vi "Loop_SM.vi"() -> ()   [LabVIEW 2017, in "Claw.lvlib"]
uses:
  Claw.lvlib
  TypeDef/CLUSTER_Two Motor Input.ctl
  <vilib>/Rock Robotics/WPI/Solenoid/WPI_SolenoidValue.ctl
  ENUM_SM_State.ctl
  TypeDef/CLUSTER_Two Motor Output.ctl
  CLUSTER_Limit_Switch_Output.ctl
  ENUM_SM_Action.ctl
  _SHARE ALL/Global Share All/Global_STOP.vi
  Global_CMD.vi
  Global_ACT Write_Data Out.vi
  Global_SM Write_Data Out.vi
panel:
  out "Solenoid Output":T1
  out "Motor Output":T2
  out "Cycle Time (S)":dbl format="%.3g"
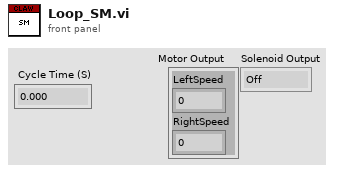
[diagram p1: front panel]
types:
  T1 = typedef "WPI_SolenoidValue.ctl" = enum16{"Off", "On", "Forward", "Reverse"}
  T2 = typedef "CLUSTER_Two Motor Input.ctl" = cluster{"LeftSpeed":dbl, "RightSpeed":dbl}
  T3 = typedef "Claw.lvlib/CLUSTER_Limit_Switch_Output.ctl" = cluster{"Limit Switch Output":bool, "Switch Pressed Count":i32}
  T4 = typedef "CLUSTER_Two Motor Output.ctl" = cluster{"LeftSpeed":dbl, "RightSpeed":dbl, "LeftCurrent":dbl, "RightCurrent":dbl}
  T5 = typedef "Claw.lvlib/ENUM_SM_State.ctl" = enum16{"Startup", "Idle", "No Cube", "Cube in Claw", "Shutdown"}
  T6 = typedef "Claw.lvlib/ENUM_SM_Action.ctl" = enum16{"No Action", "Reset Time", "Reset All", "Enable Piston", "Write Piston", "Run Motor - Free", "Run Motor - Output Only", "Disable Piston", "Increment Counter", "Reset Counter"}
  T7 = cluster{"State":T5, "Previous State":T5, "Current Time":timestamp, "Previous Time":timestamp, "Start Time":timestamp, "Target Time (ms)":u32, "Cycle Time(S)":dbl, "Motor Input":T2, "Solenoid Value: extended (t) inward (f)":bool, "Motor Output":T2, "Solenoid Output":T1, "Motor Data":T4, "Limit Switch Data":T3, "Disabled?":bool, "Max Current Value":dbl, "Current Counter":i32, "Max Counter Valve":i32}
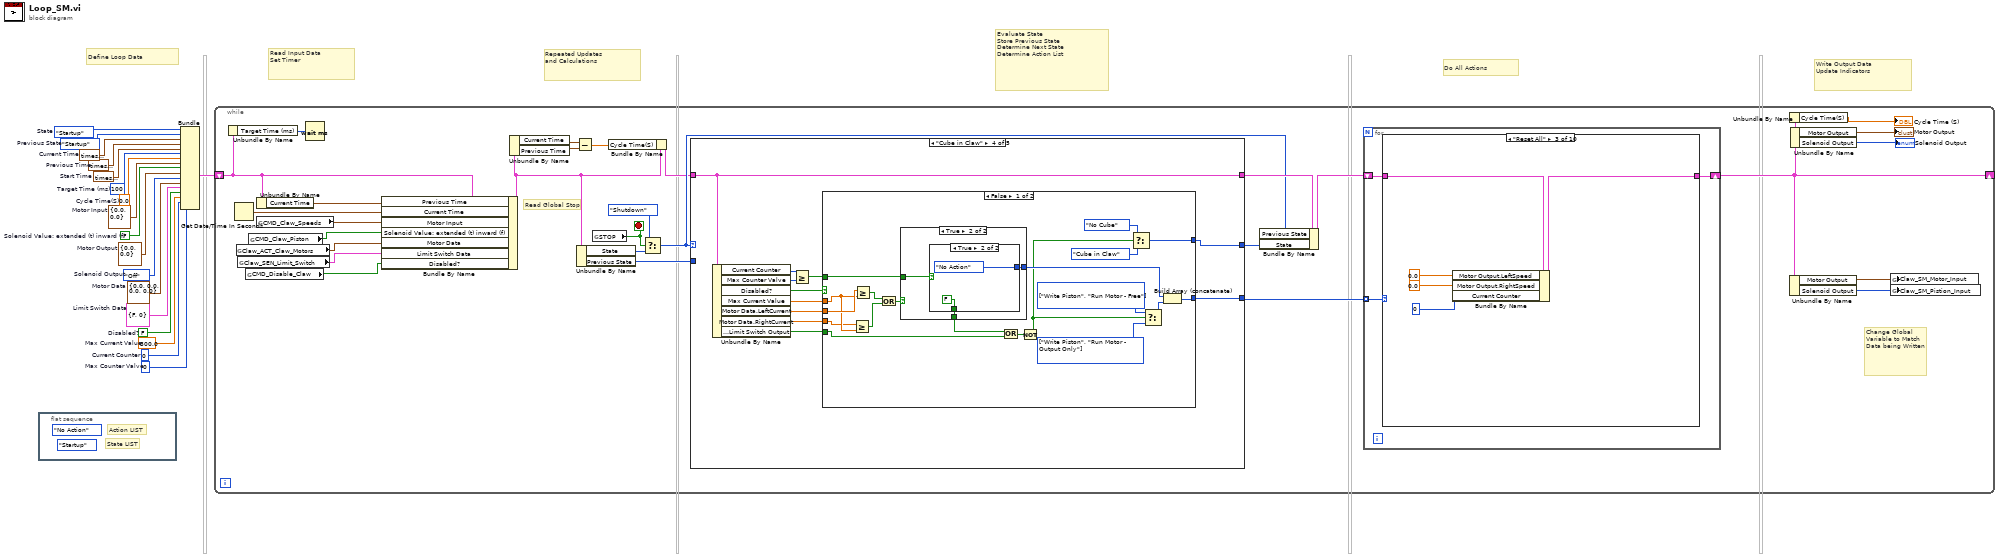
[diagram p0: block diagram]
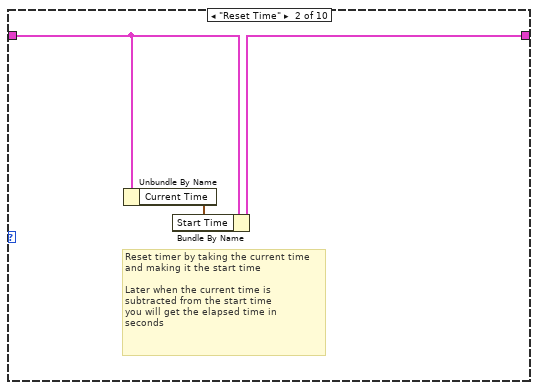
[diagram p3: hidden frame]
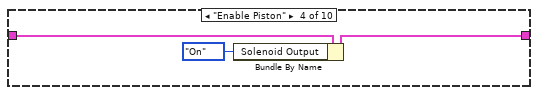
[diagram p4: hidden frame]
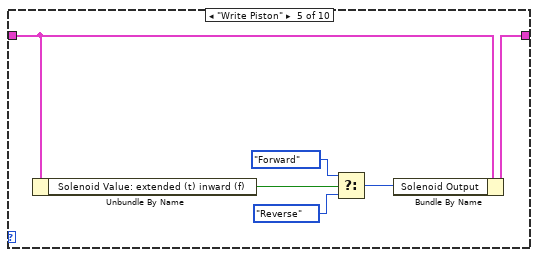
[diagram p5: hidden frame]
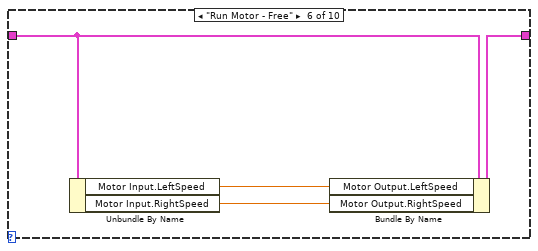
[diagram p6: hidden frame]
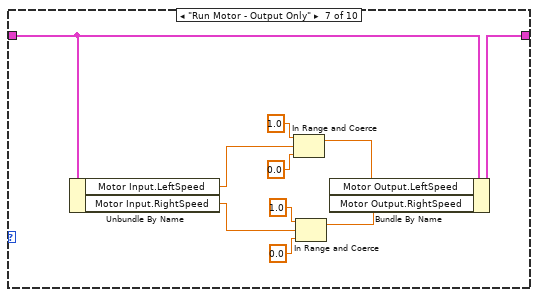
[diagram p7: hidden frame]
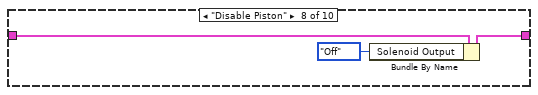
[diagram p8: hidden frame]
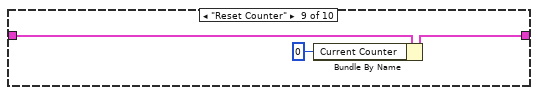
[diagram p9: hidden frame]
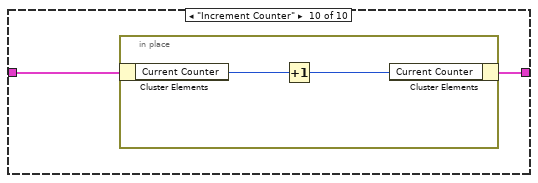
[diagram p10: hidden frame]
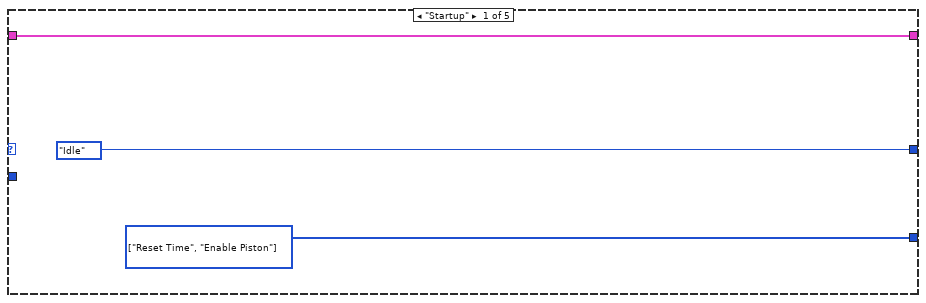
[diagram p11: hidden frame]
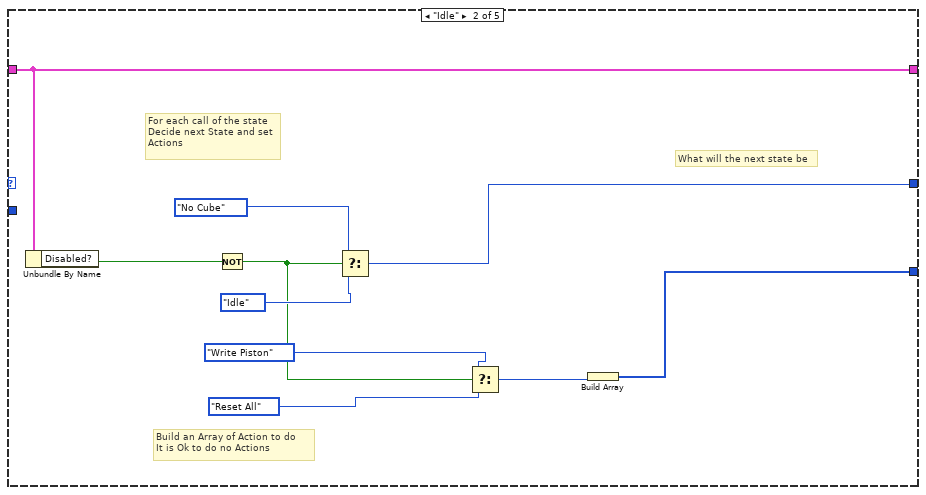
[diagram p12: hidden frame]
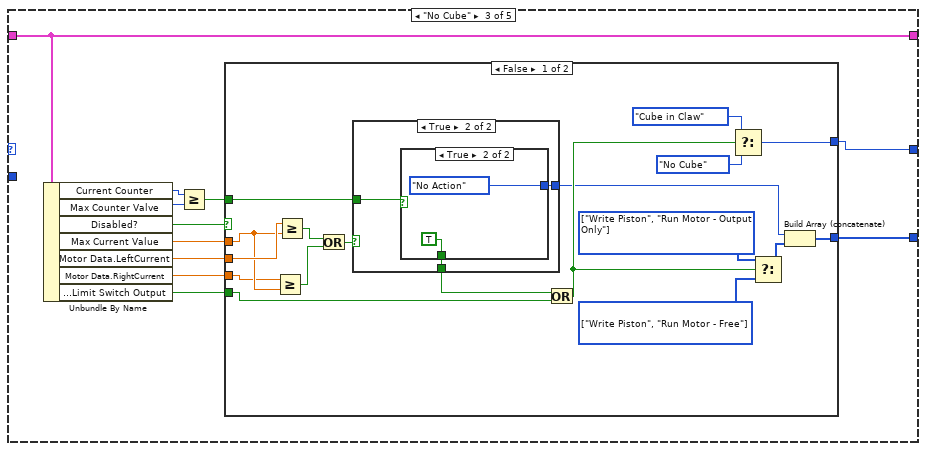
[diagram p13: hidden frame]
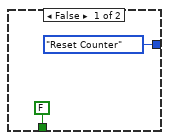
[diagram p14: hidden frame]
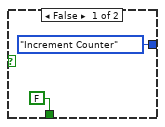
[diagram p15: hidden frame]
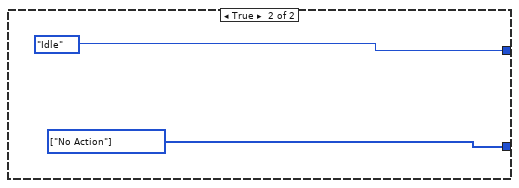
[diagram p16: hidden frame]
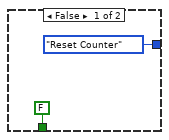
[diagram p17: hidden frame]
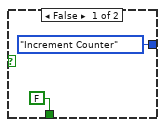
[diagram p18: hidden frame]
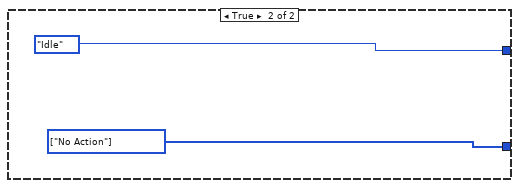
[diagram p19: hidden frame]
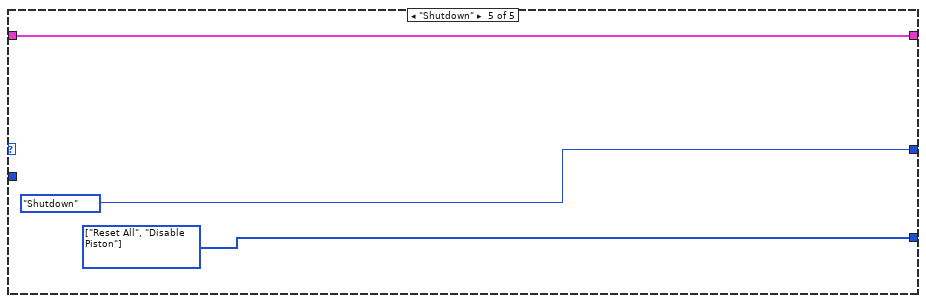
[diagram p20: hidden frame]
diagram:
  w1 = 0  # Max Counter Valve
  w2 = 0  # Current Counter
  w3 = 300.0  # Max Current Value
  w4 = FALSE  # Disabled?
  w5 = T3 {"Limit Switch Output"=FALSE, "Switch Pressed Count"=0}  # Limit Switch Data
  w6 = T4 {"LeftSpeed"=0.0, "RightSpeed"=0.0, "LeftCurrent"=0.0, "RightCurrent"=0.0}  # Motor Data
  w9 = FALSE  # Solenoid Value: extended (t) inward (f)
  w10 = T2 {"LeftSpeed"=0.0, "RightSpeed"=0.0}  # Motor Input
  w8 = T2 {"LeftSpeed"=0.0, "RightSpeed"=0.0}  # Motor Output
  w7 = WPI_SolenoidValue."Off"  # Solenoid Output
  w11 = 0.0  # Cycle Time(S)
  w12 = ENUM_SM_State."Startup"  # Previous State
  w13 = timestamp(0 s since 1904-01-01)  # Previous Time
  w14 = u32 100  # Target Time (ms)
  w15 = timestamp(0 s since 1904-01-01)  # Start Time
  w16 = timestamp(0 s since 1904-01-01)  # Current Time
  w17 = ENUM_SM_State."Startup"  # State
  # "Define Loop Data"
  # "Repeated Updates\nand Calculations"
  # "Read Input Data\nSet Timer"
  # "Evaluate State\nStore Previous State\nDetermine Next State\nDetermine Action List"
  # "Do All Actions"
  # "Write Output Data\nUpdate Indicators"
  n1 = flat-sequence {
    frame #0 {
      (unwired) ENUM_SM_State."Startup" ("State")
      (unwired) ENUM_SM_Action."No Action" ("Action")
      # "State LIST"
      # "Action LIST"
    }
  }
  n2 = Bundle("State"=w17, "Previous State"=w12, "Current Time"=w16, "Previous Time"=w13, "Start Time"=w15, "Target Time (ms)"=w14, "Cycle Time(S)"=w11, "Motor Input"=w10, "Solenoid Value: extended (t) inward (f)"=w9, "Motor Output"=w8, "Solenoid Output"=w7, "Motor Data"=w6, "Limit Switch Data"=w5, "Disabled?"=w4, "Max Current Value"=w3, "Current Counter"=w2, "Max Counter Valve"=w1) -> (w18:T7)  [unwired: 1 in]
  n3 = while {
    shift-right: [w36] -> _
    shift-left: w18 -> [w39]
    stop <- w44 stop-if-true
    # "Change Global\nVariable to Match\nData being Written"
    # "Read Global Stop"
    n4 = Unbundle By Name(w39) -> ("Target Time (ms)"=w41:u32)
    n5 = Get Date/Time In Seconds() -> (seconds since 1Jan1904=w47:timestamp)
    n6 = global read "Global_ACT Write_Data Out.vi" "Claw_ACT_Claw_Motors"() -> (w26:T4)
    n7 = global read "Global_ACT Write_Data Out.vi" "Claw_SEN_Limit_Switch"() -> (w25:T3)
    n8 = global read "Global_CMD.vi" "CMD_Disable_Claw"() -> (w24:bool)
    n9 = global read "Global_CMD.vi" "CMD_Claw_Piston"() -> (w27:bool)
    n10 = Unbundle By Name(w39) -> ("Current Time"=w40:timestamp)
    n11 = global read "Global_CMD.vi" "CMD_Claw_Speeds"() -> (w28:T2)
    n12 = Wait (ms)(milliseconds to wait=w41) -> ()  [unwired: 1 out]
    n13 = Bundle By Name(cluster=w39, "Previous Time"=w40, "Current Time"=w47, "Motor Input"=w28, "Solenoid Value: extended (t) inward (f)"=w27, "Motor Data"=w26, "Limit Switch Data"=w25, "Disabled?"=w24) -> (w32:T7)
    n14 = Unbundle By Name(w32) -> ("Current Time"=w33:timestamp, "Previous Time"=w34:timestamp)
    n15 = Subtract(x=w33, y=w34) -> (x-y=w30:dbl)
    n16 = Unbundle By Name(w32) -> ("State"=w42:T5, "Previous State"=w38:T5)
    n17 = global read "Global_STOP.vi" "STOP"() -> (w44:bool)
    n18 = Bundle By Name(cluster=w32, "Cycle Time(S)"=w30) -> (w31:T7)
    n19 = Select(t=ENUM_SM_State."Shutdown" ("State"), s=w44, f=w42) -> (s? t:f=w37:T5)
    n20 = case shown="\"Cube in Claw\"" w37 {
      tunnel: w31 -> [w95 w105 w116 w156 w189]
      tunnel: [w95 w105 w116 w156 w189] -> w45
      tunnel: [ENUM_SM_State."Idle" ("State") w104 w109 w149 ENUM_SM_State."Shutdown" ("State")] -> w23
      tunnel: [w94 w98 w110 w150 w187] -> w29
      tunnel: w38 -> [_ _ _ _ _]
      frame "Startup" {
        w94 = T6[] [enum."Reset Time", enum."Enable Piston"] items=["No Action", "Reset Time", "Reset All", "Enable Piston", "Write Piston", "Run Motor - Free", "Run Motor - Output Only", "Disable Piston", "Increment Counter", "Reset Counter"] ("Actions")
      }
      frame "Idle" {
        # "For each call of the state\nDecide next State and set\nActions"
        # "What will the next state be"
        # "Build an Array of Action to do\nIt is Ok to do no Actions"
        n21 = Unbundle By Name(w105) -> ("Disabled?"=w97:bool)
        n22 = Not(x=w97) -> (.not. x?=w96:bool)
        n23 = Select(t=ENUM_SM_State."No Cube" ("State"), s=w96, f=ENUM_SM_State."Idle" ("State")) -> (s? t:f=w104:T5)
        n24 = Select(t=ENUM_SM_Action."Write Piston" ("Action"), s=w96, f=ENUM_SM_Action."Reset All" ("Action")) -> (s? t:f=w99:T6)
        n25 = Build Array(w99) -> (w98:T6[])
      }
      frame "No Cube" {
        n26 = Unbundle By Name(w116) -> ("Current Counter"=w107:i32, "Max Counter Valve"=w108:i32, "Disabled?"=w115:bool, "Max Current Value"=w114:dbl, "Motor Data.LeftCurrent"=w113:dbl, "Motor Data.RightCurrent"=w112:dbl, "Limit Switch Data.Limit Switch Output"=w111:bool)
        n27 = Greater Or Equal?(x=w107, y=w108) -> (x >= y?=w106:bool)
        n28 = case shown="False" w115 {
          tunnel: [w123 ENUM_SM_State."Idle" ("State")] -> w109
          tunnel: w114 -> [w133 _]
          tunnel: w113 -> [w134 _]
          tunnel: w112 -> [w132 _]
          tunnel: w111 -> [w129 _]
          tunnel: [w118 w144] -> w110
          tunnel: w106 -> [w117 _]
          frame False {
            w127 = T6[] [enum."Write Piston", enum."Run Motor - Free"] items=["No Action", "Reset Time", "Reset All", "Enable Piston", "Write Piston", "Run Motor - Free", "Run Motor - Output Only", "Disable Piston", "Increment Counter", "Reset Counter"] ("Actions")
            w128 = T6[] [enum."Write Piston", enum."Run Motor - Output Only"] items=["No Action", "Reset Time", "Reset All", "Enable Piston", "Write Piston", "Run Motor - Free", "Run Motor - Output Only", "Disable Piston", "Increment Counter", "Reset Counter"] ("Actions")
            n29 = Greater Or Equal?(x=w132, y=w133) -> (x >= y?=w130:bool)
            n30 = Greater Or Equal?(x=w134, y=w133) -> (x >= y?=w131:bool)
            n31 = Or(x=w131, y=w130) -> (x .or. y?=w122:bool)
            n32 = case shown="True" w122 {
              tunnel: [FALSE w139] -> w120
              tunnel: [ENUM_SM_Action."Reset Counter" ("Action") w138] -> w119
              tunnel: w117 -> [_ w137]
              frame False {
              }
              frame True {
                n33 = case shown="True" w137 {
                  tunnel: [FALSE TRUE] -> w139
                  tunnel: [ENUM_SM_Action."Increment Counter" ("Action") ENUM_SM_Action."No Action" ("Action")] -> w138
                  frame False {
                  }
                  frame True {
                  }
                }
              }
            }
            n34 = Or(x=w120, y=w129) -> (x .or. y?=w124:bool)
            n35 = Select(t=ENUM_SM_State."Cube in Claw" ("State"), s=w124, f=ENUM_SM_State."No Cube" ("State")) -> (s? t:f=w123:T5)
            n36 = Select(t=w128, s=w124, f=w127) -> (s? t:f=w121:T6[])
            n37 = Build Array (concatenate)(w119, w121) -> (w118:T6[])
          }
          frame True {
            w144 = T6[] [enum."No Action"] items=["No Action", "Reset Time", "Reset All", "Enable Piston", "Write Piston", "Run Motor - Free", "Run Motor - Output Only", "Disable Piston", "Increment Counter", "Reset Counter"] ("Actions")
          }
        }
      }
      frame "Cube in Claw" {
        n38 = Unbundle By Name(w156) -> ("Current Counter"=w148:i32, "Max Counter Valve"=w147:i32, "Disabled?"=w155:bool, "Max Current Value"=w154:dbl, "Motor Data.LeftCurrent"=w153:dbl, "Motor Data.RightCurrent"=w152:dbl, "Limit Switch Data.Limit Switch Output"=w151:bool)
        n39 = Greater Or Equal?(x=w148, y=w147) -> (x >= y?=w146:bool)
        n40 = case shown="False" w155 {
          tunnel: [w164 ENUM_SM_State."Idle" ("State")] -> w149
          tunnel: w154 -> [w174 _]
          tunnel: w153 -> [w175 _]
          tunnel: w152 -> [w173 _]
          tunnel: w151 -> [w170 _]
          tunnel: [w159 w185] -> w150
          tunnel: w146 -> [w157 _]
          frame False {
            w168 = T6[] [enum."Write Piston", enum."Run Motor - Output Only"] items=["No Action", "Reset Time", "Reset All", "Enable Piston", "Write Piston", "Run Motor - Free", "Run Motor - Output Only", "Disable Piston", "Increment Counter", "Reset Counter"] ("Actions")
            w169 = T6[] [enum."Write Piston", enum."Run Motor - Free"] items=["No Action", "Reset Time", "Reset All", "Enable Piston", "Write Piston", "Run Motor - Free", "Run Motor - Output Only", "Disable Piston", "Increment Counter", "Reset Counter"] ("Actions")
            n41 = Greater Or Equal?(x=w173, y=w174) -> (x >= y?=w171:bool)
            n42 = Greater Or Equal?(x=w175, y=w174) -> (x >= y?=w172:bool)
            n43 = Or(x=w172, y=w171) -> (x .or. y?=w163:bool)
            n44 = case shown="True" w163 {
              tunnel: [FALSE w180] -> w161
              tunnel: [ENUM_SM_Action."Reset Counter" ("Action") w179] -> w160
              tunnel: w157 -> [_ w178]
              frame False {
              }
              frame True {
                n45 = case shown="True" w178 {
                  tunnel: [FALSE FALSE] -> w180
                  tunnel: [ENUM_SM_Action."Increment Counter" ("Action") ENUM_SM_Action."No Action" ("Action")] -> w179
                  frame False {
                  }
                  frame True {
                  }
                }
              }
            }
            n46 = Or(x=w161, y=w170) -> (x .or. y?=w165:bool)
            n47 = Not(x=w165) -> (.not. x?=w158:bool)
            n48 = Select(t=ENUM_SM_State."No Cube" ("State"), s=w158, f=ENUM_SM_State."Cube in Claw" ("State")) -> (s? t:f=w164:T5)
            n49 = Select(t=w169, s=w158, f=w168) -> (s? t:f=w162:T6[])
            n50 = Build Array (concatenate)(w160, w162) -> (w159:T6[])
          }
          frame True {
            w185 = T6[] [enum."No Action"] items=["No Action", "Reset Time", "Reset All", "Enable Piston", "Write Piston", "Run Motor - Free", "Run Motor - Output Only", "Disable Piston", "Increment Counter", "Reset Counter"] ("Actions")
          }
        }
      }
      frame "Shutdown" {
        w187 = T6[] [enum."Reset All", enum."Disable Piston"] items=["No Action", "Reset Time", "Reset All", "Enable Piston", "Write Piston", "Run Motor - Free", "Run Motor - Output Only", "Disable Piston", "Increment Counter", "Reset Counter"] ("Actions")
      }
    }
    n51 = Bundle By Name(cluster=w45, "Previous State"=w37, "State"=w23) -> (w46:T7)
    n52 = for {
      tunnel: w29 -> [w50] mode=indexing
      shift-right: [w49] -> w36
      shift-left: w46 -> [w48]
      n53 = case shown="\"Reset All\"" w50 {
        tunnel: w48 -> [w51 w54 w59 w62 w68 w72 w82 w85 w88 w90]
        tunnel: [w51 w53 w58 w61 w67 w71 w81 w84 w87 w89] -> w49
        frame "No Action" {
        }
        frame "Reset Time" {
          # "Reset timer by taking the current time\nand making it the start time\n\nLater when the current time is \nsubtracted from the start time\nyou will get the elapsed time in \nseconds"
          n54 = Unbundle By Name(w54) -> ("Current Time"=w52:timestamp)
          n55 = Bundle By Name(cluster=w54, "Start Time"=w52) -> (w53:T7)
        }
        frame "Reset All" {
          n56 = Bundle By Name(cluster=w59, "Motor Output.LeftSpeed"=0.0, "Motor Output.RightSpeed"=0.0, "Current Counter"=0) -> (w58:T7)
        }
        frame "Enable Piston" {
          n57 = Bundle By Name(cluster=w62, "Solenoid Output"=WPI_SolenoidValue."On") -> (w61:T7)
        }
        frame "Write Piston" {
          n58 = Unbundle By Name(w68) -> ("Solenoid Value: extended (t) inward (f)"=w66:bool)
          n59 = Select(t=WPI_SolenoidValue."Forward" ("Solenoid Output"), s=w66, f=WPI_SolenoidValue."Reverse" ("Solenoid Output")) -> (s? t:f=w63:T1)
          n60 = Bundle By Name(cluster=w68, "Solenoid Output"=w63) -> (w67:T7)
        }
        frame "Run Motor - Free" {
          n61 = Unbundle By Name(w72) -> ("Motor Input.LeftSpeed"=w70:dbl, "Motor Input.RightSpeed"=w69:dbl)
          n62 = Bundle By Name(cluster=w72, "Motor Output.LeftSpeed"=w70, "Motor Output.RightSpeed"=w69) -> (w71:T7)
        }
        frame "Run Motor - Output Only" {
          n63 = Unbundle By Name(w82) -> ("Motor Input.LeftSpeed"=w78:dbl, "Motor Input.RightSpeed"=w74:dbl)
          n64 = In Range and Coerce(upper limit=1.0, x=w78, lower limit=0.0) -> (coerced(x)=w77:dbl)  [unwired: 1 out]
          n65 = In Range and Coerce(upper limit=1.0, x=w74, lower limit=0.0) -> (coerced(x)=w73:dbl)  [unwired: 1 out]
          n66 = Bundle By Name(cluster=w82, "Motor Output.LeftSpeed"=w77, "Motor Output.RightSpeed"=w73) -> (w81:T7)
        }
        frame "Disable Piston" {
          n67 = Bundle By Name(cluster=w85, "Solenoid Output"=WPI_SolenoidValue."Off") -> (w84:T7)
        }
        frame "Reset Counter" {
          n68 = Bundle By Name(cluster=w88, "Current Counter"=0) -> (w87:T7)
        }
        frame "Increment Counter" {
          n69 = in-place {
            n70 = in-place-cluster #1(w90) -> ("Current Counter"=w92:i32)
            n71 = Increment(x=w92) -> (x+1=w91:i32)
            n72 = in-place-cluster #1("Current Counter"=w91) -> (w89:T7)
          }
        }
      }
    }
    n73 = Unbundle By Name(w36) -> ("Cycle Time(S)"=→"Cycle Time (S)":dbl)
    n74 = Unbundle By Name(w36) -> ("Motor Output"=w21:T2, "Solenoid Output"=w22:T1)
    n75 = Unbundle By Name(w36) -> ("Motor Output"=→"Motor Output":T2, "Solenoid Output"=→"Solenoid Output":T1)
    n76 = global write "Global_SM Write_Data Out.vi" "Claw_SM_Motor_Input"(w21) -> ()
    n77 = global write "Global_SM Write_Data Out.vi" "Claw_SM_Pistion_Input"(w22) -> ()
  }
